vi "Load Details.vi"(8 "error in (no error)":errorcluster, 11 "Alarms":path) -> (0 "error out":errorcluster, 3 "Alarms Details":T1[](array[typedef]))   [LabVIEW 2015, in "Alarm Handler Actor.lvclass"]
doc: "Loads the Alarms Details information from the specified <b>Alarms</b> file."
uses:
  Alarm Handler Actor.lvclass
  Alarm Details.ctl
panel:
  out "subarray":string[][](array[string])
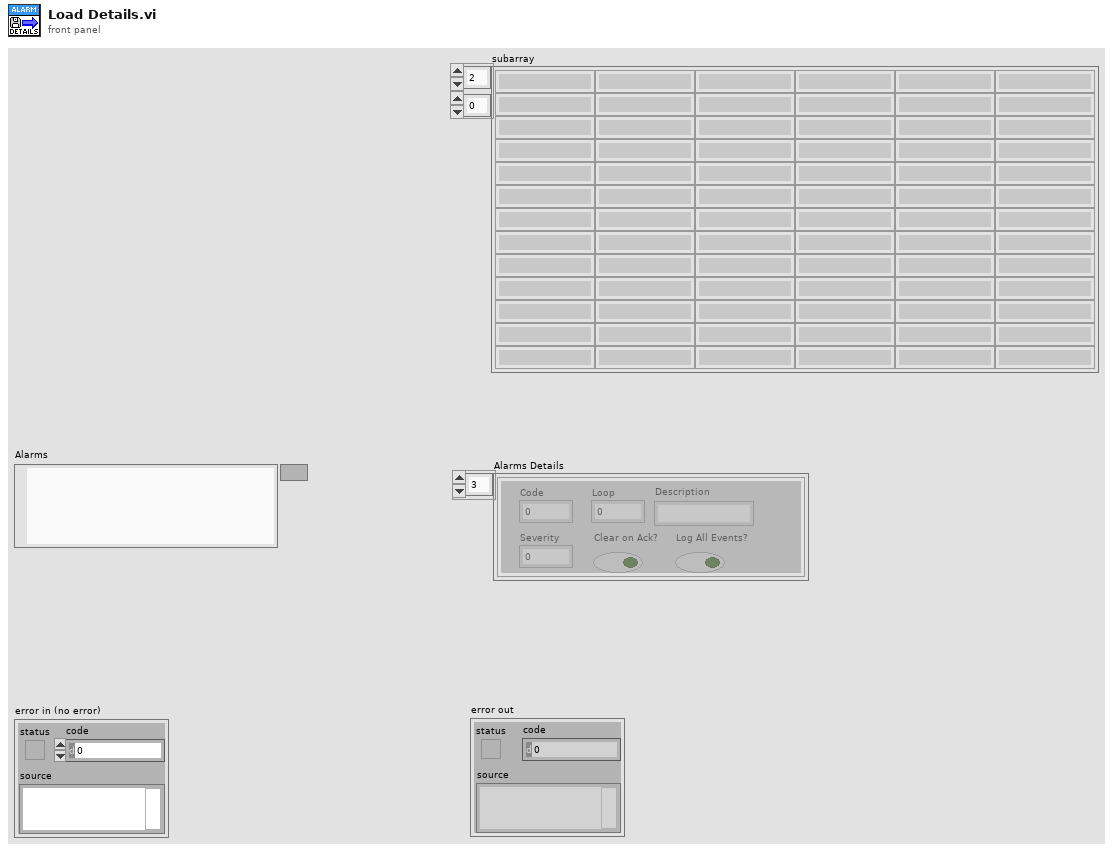
[diagram p1: front panel]
types:
  T1 = typedef "Alarm Handler Actor.lvclass/Alarm Details.ctl" = cluster{"Code":i32, "Loop":i32, "Description":string, "Severity":i32, "Clear on Ack?":bool, "Log All Events?":bool}
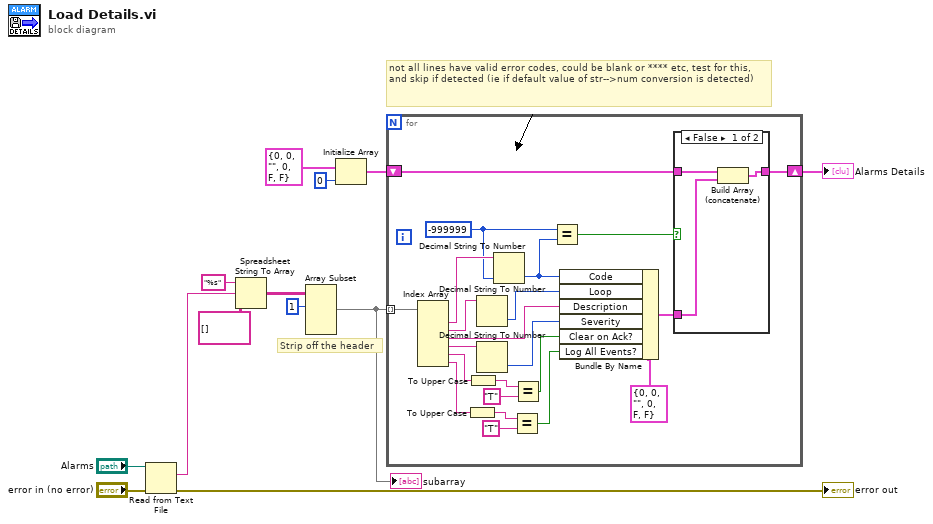
[diagram p0: block diagram]
diagram:
  # "not all lines have valid error codes, could be blank or **** etc, test for this, and skip if detected (ie if default value of str-->num conversion is detected)"
  # "Strip off the header"
  n1 = Read from Text File(file (use dialog)="Alarms", error in="error in (no error)") -> (text=w10:string, error out=→"error out":errorcluster)  [unwired: 4 out]
  n2 = Spreadsheet String To Array(format string="%s", spreadsheet string=w10, array type (2D Dbl)=string[][] []) -> (array=w5:string[][])  [unwired: 1 out]
  n3 = Array Subset(array=w5, index (row)=1 ("index")) -> (w4:string[][])  [unwired: 3 in]
  "subarray" <- w4
  n4 = Initialize Array(T1 {"Code"=0, "Loop"=0, "Description"="", "Severity"=0, "Clear on Ack?"=FALSE, "Log All Events?"=FALSE} ("Error Detail"), 0 ("dimension size")) -> (w6:T1[])
  n5 = for {
    tunnel: w4 -> [w35] mode=indexing
    shift-right: [w23] -> w1
    shift-left: w6 -> [w25]
    w21 = -999999 ("default (0 I32)")
    n6 = Index Array(array=w35) -> (element #1=w22:string, element #2=w34:string, element #3=w26:string, element #4=w32:string, element #5=w29:string, element #6=w16:string)  [unwired: 6 in]
    n7 = To Upper Case(1:w16) -> (0:w19:string)
    n8 = To Upper Case(1:w29) -> (0:w28:string)
    n9 = Decimal String To Number(string=w34) -> (number=w33:i32)  [unwired: 3 out]
    n10 = Decimal String To Number(string=w32) -> (number=w31:i32)  [unwired: 3 out]
    n11 = Decimal String To Number(string=w22, default (0L)=w21) -> (number=w15:i32)  [unwired: 2 out]
    n12 = Equal?(x=w19, y="T") -> (x = y?=w17:bool)
    n13 = Equal?(x=w28, y="T") -> (x = y?=w27:bool)
    n14 = Equal?(x=w21, y=w15) -> (x = y?=w20:bool)
    n15 = Bundle By Name(cluster=T1 {"Code"=0, "Loop"=0, "Description"="", "Severity"=0, "Clear on Ack?"=FALSE, "Log All Events?"=FALSE} ("Error Detail"), "Code"=w15, "Loop"=w33, "Description"=w26, "Severity"=w31, "Clear on Ack?"=w27, "Log All Events?"=w17) -> (w24:T1)
    n16 = case shown="False" w20 {
      tunnel: w25 -> [w38 w39]
      tunnel: w24 -> [w37 _]
      tunnel: [w36 w39] -> w23
      frame False {
        n17 = Build Array (concatenate)(w38, w37) -> (w36:T1[])
      }
      frame True {
      }
    }
  }
  "Alarms Details" <- w1
